vi "质控启动参数选择对话框.vi"() -> (1 "取消启动":bool, 2 "确定启动":bool, 3 "启动模块":T1)   [LabVIEW 2016, in "质控单元.lvlib"]
panel:
  in  "总氮":bool
  in  "确定":bool
  in  "COD":bool
  in  "总磷":bool
  in  "取消":bool
  in  "氨氮":bool
  # "请选择加标回收模块"
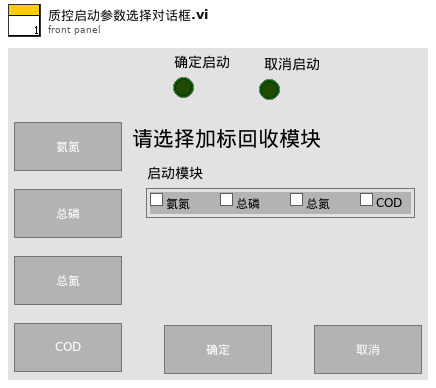
[diagram p1: front panel]
types:
  T1 = cluster{"氨氮":bool, "总磷":bool, "总氮":bool, "COD":bool}
  T2 = cluster{"氨氮1":bool, "总磷1":bool, " COD1":bool, "总磷1 2":bool}
  T3 = cluster{"氨氮1":bool, "总磷1":bool, "总氮":bool, " COD1":bool}
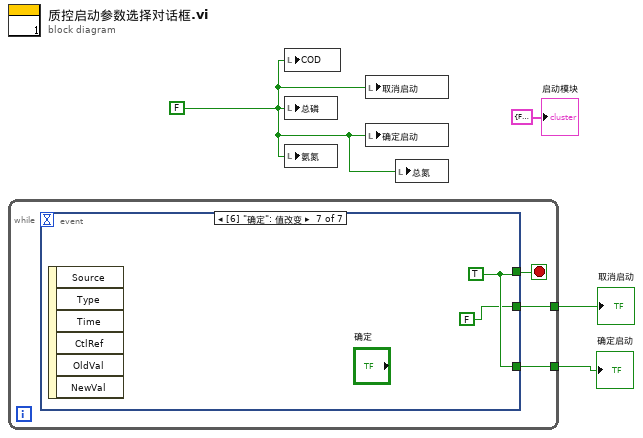
[diagram p0: block diagram]
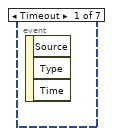
[diagram p2: hidden frame]
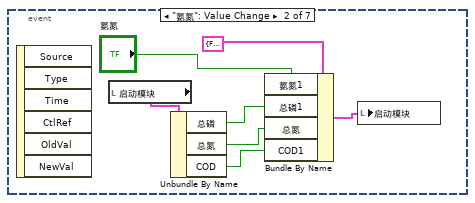
[diagram p3: hidden frame]
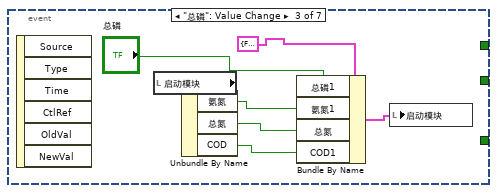
[diagram p4: hidden frame]
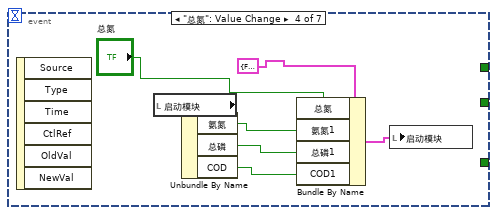
[diagram p5: hidden frame]
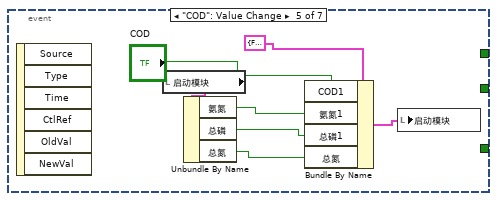
[diagram p6: hidden frame]
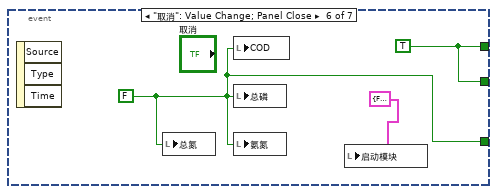
[diagram p7: hidden frame]
diagram:
  w1 = FALSE ("确定")
  n1 = while {
    tunnel: [w6] -> w4
    tunnel: [w5] -> w3
    stop <- w7 stop-if-true
    n2 = event shown="[6] \"确定\": 值改变" {
      selector: _ -> [_ _ _ _ _ _ _]
      dyn-events: _ -> [_ _ _ _ _ _ _]
      timeout: _ -> [_ _ _ _ _ _ _]
      tunnel: [_ _ _ _ _ w38 w40] -> w7
      tunnel: [_ _ _ _ _ w36 w40] -> w6
      tunnel: [_ _ _ _ _ w38 FALSE ("确定")] -> w5
      event Timeout {
        n3 = event-data() -> ()  [unwired: 1 in, 3 out]
      }
      event "氨氮": Value Change {
        n4 = event-data() -> ()  [unwired: 1 in, 6 out]
        n5 = local read "启动模块"() -> (w13:T1)
        n6 = Unbundle By Name(w13) -> ("总磷"=w12:bool, "总氮"=w11:bool, "COD"=w9:bool)
        n7 = Bundle By Name(cluster=T3 {"氨氮1"=FALSE, "总磷1"=FALSE, "总氮"=FALSE, " COD1"=FALSE} ("启动模块"), "氨氮1"="氨氮", "总磷1"=w12, "总氮"=w11, "COD1"=w9) -> (w8:T3)
        n8 = local write "启动模块"(w8) -> ()
      }
      event "总磷": Value Change {
        n9 = event-data() -> ()  [unwired: 1 in, 6 out]
        n10 = local read "启动模块"() -> (w21:T1)
        n11 = Unbundle By Name(w21) -> ("氨氮"=w20:bool, "总氮"=w19:bool, "COD"=w15:bool)
        n12 = Bundle By Name(cluster=T3 {"氨氮1"=FALSE, "总磷1"=FALSE, "总氮"=FALSE, " COD1"=FALSE} ("启动模块"), "总磷1"="总磷", "氨氮1"=w20, "总氮"=w19, "COD1"=w15) -> (w18:T3)
        n13 = local write "启动模块"(w18) -> ()
      }
      event "总氮": Value Change {
        n14 = event-data() -> ()  [unwired: 1 in, 6 out]
        n15 = local read "启动模块"() -> (w28:T1)
        n16 = Unbundle By Name(w28) -> ("氨氮"=w27:bool, "总磷"=w26:bool, "COD"=w23:bool)
        n17 = Bundle By Name(cluster=T3 {"氨氮1"=FALSE, "总磷1"=FALSE, "总氮"=FALSE, " COD1"=FALSE} ("启动模块"), "总氮"="总氮", "氨氮1"=w27, "总磷1"=w26, "COD1"=w23) -> (w25:T3)
        n18 = local write "启动模块"(w25) -> ()
      }
      event "COD": Value Change {
        n19 = event-data() -> ()  [unwired: 1 in, 6 out]
        n20 = local read "启动模块"() -> (w35:T1)
        n21 = Unbundle By Name(w35) -> ("氨氮"=w34:bool, "总磷"=w33:bool, "总氮"=w29:bool)
        n22 = Bundle By Name(cluster=T3 {"氨氮1"=FALSE, "总磷1"=FALSE, "总氮"=FALSE, " COD1"=FALSE} ("启动模块"), "COD1"="COD", "氨氮1"=w34, "总磷1"=w33, "总氮"=w29) -> (w32:T3)
        n23 = local write "启动模块"(w32) -> ()
      }
      event "取消": Value Change; Panel Close {
        w36 = FALSE ("确定")
        w38 = TRUE ("确定")
        n24 = event-data() -> ()  [unwired: 1 in, 3 out]
        n25 = local write "总氮"(w36) -> ()
        n26 = local write "COD"(w36) -> ()
        n27 = local write "总磷"(w36) -> ()
        n28 = local write "氨氮"(w36) -> ()
        n29 = local write "启动模块"(T2 {"氨氮1"=FALSE, "总磷1"=FALSE, " COD1"=FALSE, "总磷1 2"=FALSE} ("启动模块")) -> ()
      }
      event "确定": Value Change {
        w40 = TRUE ("确定")
        n30 = event-data() -> ()  [unwired: 1 in, 6 out]
      }
    }
  }
  "确定启动" <- w4
  "取消启动" <- w3
  n31 = local write "COD"(w1) -> ()
  n32 = local write "总磷"(w1) -> ()
  n33 = local write "氨氮"(w1) -> ()
  n34 = local write "取消启动"(w1) -> ()
  n35 = local write "确定启动"(w1) -> ()
  n36 = local write "总氮"(w1) -> ()
  "启动模块" <- T2 {"氨氮1"=FALSE, "总磷1"=FALSE, " COD1"=FALSE, "总磷1 2"=FALSE} ("启动模块")
